vi "SIGGEN_AMPL.vi"(0 "Session In":refnum<visa-resource-name>="GPIB0::18::INSTR", 2 "Skip(T)":bool, 5 "Max Power":dbl=20.0, 7 "OFFS_IN":dbl, 9 "Set Power (num)":dbl=-25.0, 11 "error in":errorcluster {"code" format="%.0x"}, 12 "RO(T)":bool, 14 "delay after set (ms)":i32 caption="Delay Time (s)") -> (4 "Session Out":refnum<visa-resource-name>="GPIB0::18::INSTR", 6 "OFFS_OUT":dbl=-25.0, 10 "Get Power":dbl=-25.0, 15 "error out":errorcluster {"code" format="%.0x"})   [LabVIEW 2018]
doc: "Set/Get the ESG RF Amplitude in current units."
uses:
  <vilib>/Utility/error.llb/DialogType.ctl
panel:
  in  "Timeout":u32=3000
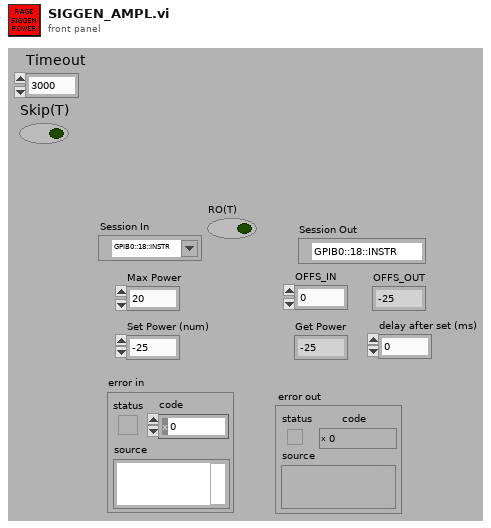
[diagram p1: front panel]
types:
  T1 = typedef "DialogType.ctl" = u16
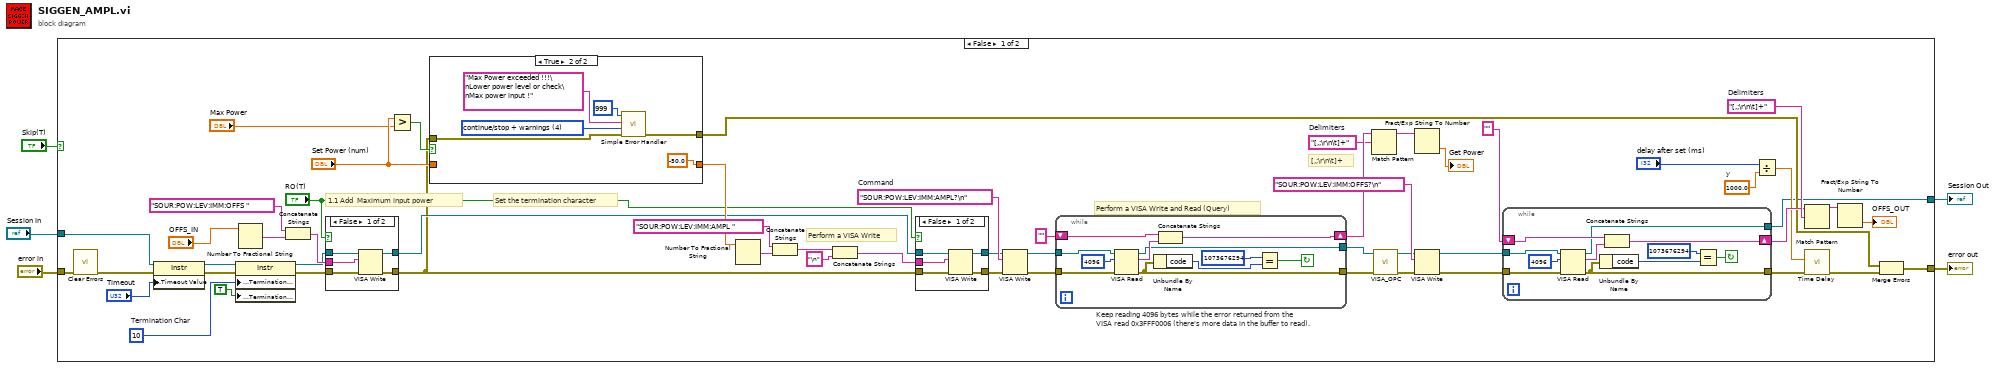
[diagram p0: block diagram]
diagram:
  n1 = case shown="False" "Skip(T)" {
    tunnel: "Session In" -> [w60 w107]
    tunnel: "error in" -> [w22 w106]
    tunnel: [w7 w106] -> w3
    tunnel: [w6 w107] -> w2
    frame False {
      w12 = 1000.0  # y
      w32 = "[,;\r\n\t]+"  # Delimiters
      w45 = "[,;\r\n\t]+"  # Delimiters
      w46 = "SOUR:POW:LEV:IMM:AMPL?\n"  # Command
      w57 = u8 10  # Termination Char
      # "1.1 Add  Maximum input power"
      # "[,;\\r\\n\\t]+"
      # "Perform a VISA Write and Read (Query)"
      # "Keep reading 4096 bytes while the error returned from the\nVISA read 0x3FFF0006 (there's more data in the buffer to read)."
      # "Perform a VISA Write"
      # "Set the termination character"
      n2 = call <vilib>:"Clear Errors.vi"("error in (no error)"=w22) -> ("error out"=w8:errorcluster)  [unwired: 5 in, 1 out]
      n3 = property class="Instr"(reference=w60, error in=w8, "General Settings:Timeout Value"="Timeout") -> (reference out=w59:refnum<visa-resource-name>, error out=w58:errorcluster)
      n4 = property class="Instr"(reference=w59, error in=w58, "Message Based Settings:Termination Character"=w57, "Message Based Settings:Termination Character Enable"=TRUE ("enable")) -> (reference out=w20:refnum<visa-resource-name>, error out=w21:errorcluster)
      n5 = Number To Fractional String(number="OFFS_IN") -> (F-format string=w38:string)  [unwired: 3 in]
      n6 = Concatenate Strings("SOUR:POW:LEV:IMM:OFFS " ("staticText"), w38) -> (w30:string)
      n7 = case shown="False" "RO(T)" {
        tunnel: w30 -> [w66 _]
        tunnel: w21 -> [w65 w68]
        tunnel: [w64 w68] -> w11
        tunnel: w20 -> [w62 w67]
        tunnel: [w63 w67] -> w19
        frame False {
          n8 = VISA Write(VISA resource name=w62, write buffer=w66, error in (no error)=w65) -> (VISA resource name out=w63:refnum<visa-resource-name>, error out=w64:errorcluster)  [unwired: 1 out]
        }
        frame True {
        }
      }
      n9 = Greater?(x="Set Power (num)", y="Max Power") -> (0:w39:bool)
      n10 = case shown="True" w39 {
        tunnel: [w88 -50.0] -> w43
        tunnel: "Set Power (num)" -> [w88 _]
        tunnel: w11 -> [w87 w93]
        tunnel: [w87 w92] -> w10
        frame False {
        }
        frame True {
          w89 = T1 4 items=["no dialog", "OK message", "continue or stop message", "OK message + warnings", "continue/stop + warnings"] ("type of dialog (OK msg:1)")
          n11 = call <vilib>:"Simple Error Handler.vi"("error code (no error:0)"=999, "error source (\" \")"="Max Power exceeded !!!\nLower power level or check\nMax power input !" ("error source (\" \")"), "type of dialog (OK msg:1)"=w89, "error in (no error)"=w93) -> ("error out"=w92:errorcluster)  [unwired: 1 in, 4 out]
        }
      }
      n12 = Number To Fractional String(number=w43) -> (F-format string=w44:string)  [unwired: 3 in]
      n13 = Concatenate Strings("SOUR:POW:LEV:IMM:AMPL " ("staticText"), w44) -> (w55:string)
      n14 = Concatenate Strings(w55, "\n" ("StaticText")) -> (w53:string)
      n15 = case shown="False" "RO(T)" {
        tunnel: w11 -> [w84 w86]
        tunnel: [w81 w86] -> w29
        tunnel: w53 -> [w83 _]
        tunnel: w19 -> [w82 w85]
        tunnel: [w80 w85] -> w18
        frame False {
          n16 = VISA Write(VISA resource name=w82, write buffer=w83, error in (no error)=w84) -> (VISA resource name out=w80:refnum<visa-resource-name>, error out=w81:errorcluster)  [unwired: 1 out]
        }
        frame True {
        }
      }
      n17 = VISA Write(VISA resource name=w18, write buffer=w46, error in (no error)=w29) -> (VISA resource name out=w51:refnum<visa-resource-name>, error out=w49:errorcluster)  [unwired: 1 out]
      n18 = while {
        tunnel: w51 -> [w102]
        shift-right: [w96] -> w50
        shift-left: "" -> [w101]
        tunnel: w49 -> [w99]
        tunnel: [w98] -> w48
        tunnel: [w95] -> w16
        stop <- w97 continue-if-true
        n19 = VISA Read(VISA resource name=w102, byte count=u32 4096 ("byte count (0)"), error in (no error)=w99) -> (VISA resource name out=w95:refnum<visa-resource-name>, read buffer=w100:string, error out=w98:errorcluster)  [unwired: 1 out]
        n20 = Unbundle By Name(w98) -> ("code"=w104:i32)
        n21 = Concatenate Strings(w101, w100) -> (w96:string)
        n22 = Equal?(x=1073676294, y=w104) -> (x = y?=w97:bool)
      }
      n23 = Match Pattern(string=w50, regular expression=w45) -> (before substring=w42:string)  [unwired: 1 in, 3 out]
      n24 = call "VISA_OPC.vi"("error in"=w48, "Session In"=w16) -> ("error out"=w17:errorcluster, "Session Out"=w15:refnum<visa-resource-name>)  [unwired: 7 in, 1 out]
      n25 = Fract/Exp String To Number(string=w42) -> (number=→"Get Power":dbl)  [unwired: 3 in, 1 out]
      n26 = VISA Write(VISA resource name=w15, write buffer="SOUR:POW:LEV:IMM:OFFS?\n" ("staticText"), error in (no error)=w17) -> (VISA resource name out=w23:refnum<visa-resource-name>, error out=w25:errorcluster)  [unwired: 1 out]
      n27 = while {
        tunnel: w23 -> [w76]
        shift-right: [w70] -> w31
        shift-left: "" -> [w75]
        tunnel: w25 -> [w73]
        tunnel: [w72] -> w28
        tunnel: [w69] -> w6
        stop <- w71 continue-if-true
        n28 = VISA Read(VISA resource name=w76, byte count=u32 4096 ("byte count (0)"), error in (no error)=w73) -> (VISA resource name out=w69:refnum<visa-resource-name>, read buffer=w74:string, error out=w72:errorcluster)  [unwired: 1 out]
        n29 = Unbundle By Name(w72) -> ("code"=w78:i32)
        n30 = Concatenate Strings(w75, w74) -> (w70:string)
        n31 = Equal?(x=1073676294, y=w78) -> (x = y?=w71:bool)
      }
      n32 = Divide(x="delay after set (ms)", y=w12) -> (x/y=w13:dbl)
      n33 = Match Pattern(string=w31, regular expression=w32) -> (before substring=w34:string)  [unwired: 1 in, 3 out]
      n34 = call "Time Delay"("error in (no error)"=w28, "Delay Time (s)"=w13) -> ("error out"=w9:errorcluster)  [unwired: 9 in]
      n35 = Fract/Exp String To Number(string=w34) -> (number=→"OFFS_OUT":dbl)  [unwired: 3 in, 1 out]
      n36 = Merge Errors(w10, w9) -> (w7:errorcluster)
    }
    frame True {
    }
  }
  "error out" <- w3
  "Session Out" <- w2
